vi "LabvolutionSubmoduleCheck_StandardOutputCallback.vi"(4 "Standard Output":refnum<user-event>, 5 "Event Data":cluster{"data":string}, 6 "Control Ref":refnum<k24>, 7 "Event Common Data":T1) -> ()   [LabVIEW 2018]
uses:
  C:/Users/GregPayne/Documents/grp/personal/labvolution-submodule-check/LabvolutionSubmoduleCheck/SystemExec.dll
  SystemExec.dll
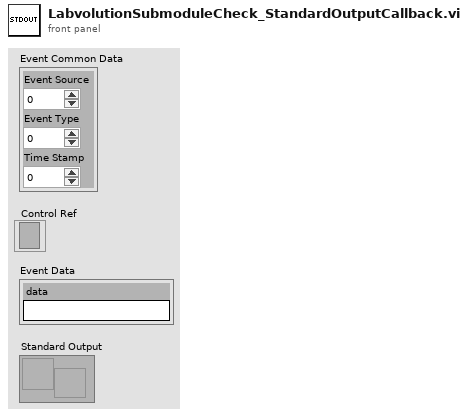
[diagram p1: front panel]
types:
  T1 = cluster{"Event Source":i32, "Event Type":u32, "Time Stamp":u32}
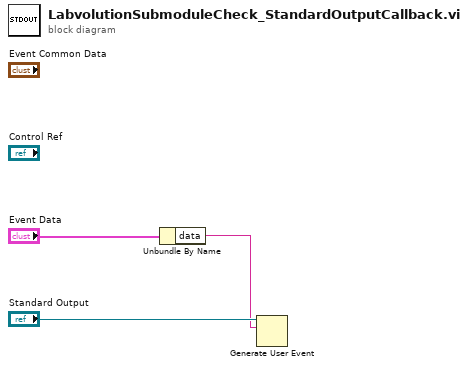
[diagram p0: block diagram]
diagram:
  n1 = Unbundle By Name("Event Data") -> ("data"=w1:string)
  n2 = Generate User Event(user event="Standard Output", event data cluster=w1) -> ()  [unwired: 2 in, 2 out]
